vi "Vision Auto Target.vi"(11 "navX Device":T1={"Interface"={"Protocol"=enum."SERIAL", "Update Rate (4Hz-60Hz)"=4, "navX Open TypeDef"=variant}, "Notify Packet"=refnum, "Loop VI Refnum"=refnum, "Ready to Close Occurrence Refnum"=refnum} {"Interface"."Update Rate (4Hz-60Hz)" min=4 max=60 step=1}) -> ()   [LabVIEW 2015]
uses:
  NavX/navX Library v2/TypeDefs/Z900_navX_DeviceTypeDef.ctl
  NavX/navX Library v2/TypeDefs/Z900_navX_ProtocolTypeDef.ctl
  NavX/navX Library v2/TypeDefs/Z900_navX_NotifyPacketTypeDef.ctl
  NavX/navX Library v2/TypeDefs/Z900_navX_ActionTypeDef.ctl
  Team Code/Robot Global Data.vi
  <vilib>/Rock Robotics/Network Tables/NT Write Number.vi
  NavX/navX Library v2/navX Library v2.lvlib
panel:
  in  "Vertical Linear Relationship":dbl
  out "VisionVertical":cluster{"VisionGyroTarget":dbl, dbl, dbl}(graph)
  out "VisionStateDistance":enum16{"Disabled", "Enable", "Suspended", "PID"}(ring)
  in  "VeriticalOffset":dbl=0.033
  in  "Y gain":dbl=80.0
  in  "minimumVisionValue":dbl=0.45
  in  "X Gain":dbl=80.0
  in  "minimumVisionValue":dbl=0.45
  out "VisionHorizontal":cluster{"VisionGyroTarget":dbl, dbl, dbl}(graph)
  out "VisionStateAngle":enum16{"Disabled", "Enable", "Suspended", "PID"}(ring)
  in  "HorizontalOffset":dbl=0.066
  # "More positive = counter clockwise\nMore negative = clockwise"
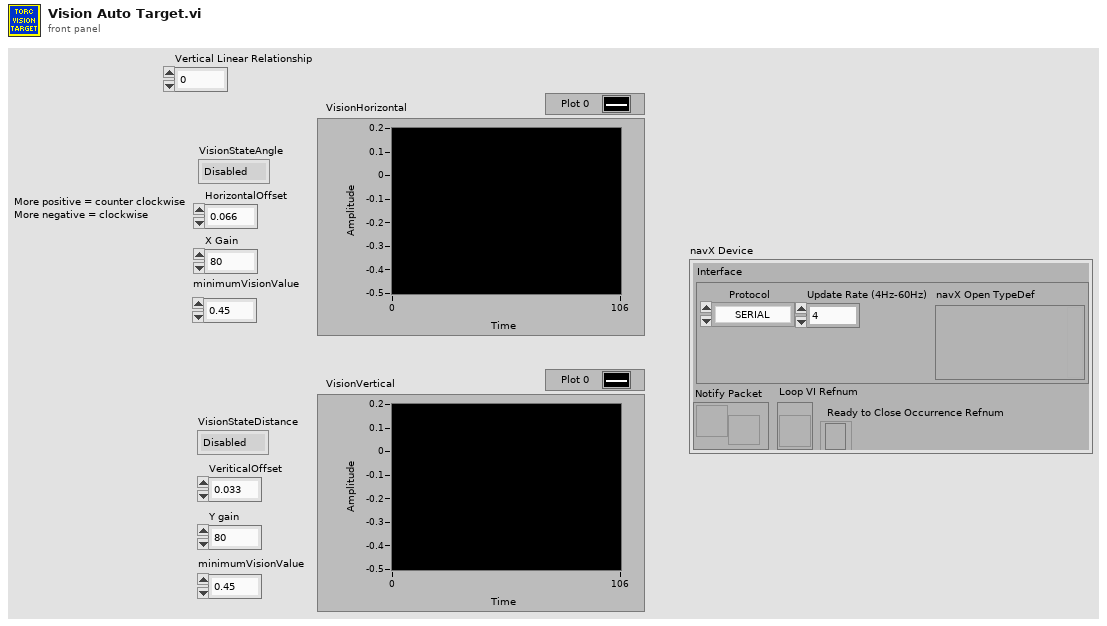
[diagram p1: front panel]
types:
  T1 = typedef "navX Library v2.lvlib/Z900_navX_DeviceTypeDef.ctl" = cluster{"Interface":cluster{"Protocol":T2, "Update Rate (4Hz-60Hz)":u8, "navX Open TypeDef":variant}, "Notify Packet":refnum<notifier>, "Loop VI Refnum":refnum<vi>, "Ready to Close Occurrence Refnum":refnum<k4>}
  T2 = typedef "navX Library v2.lvlib/Z900_navX_ProtocolTypeDef.ctl" = enum16{"SERIAL", "I2C", "SPI"}
  T3 = cluster{"Yaw":dbl, "Roll":dbl, "Pitch":dbl, "Heading":dbl, "Fused Heading":dbl}
  T4 = cluster{"Distance (ft)":dbl, "Center":cluster{dbl, dbl}, "Normalized Rect":cluster{"Numeric":dbl, "Numeric 2":dbl, "Numeric 3":dbl, "Numeric 5":dbl}}[]
  T5 = cluster{"Detected Targets[0]":cluster{"Distance (ft)":dbl, "Center":cluster{dbl, dbl}, "Normalized Rect":cluster{"Numeric":dbl, "Numeric 2":dbl, "Numeric 3":dbl, "Numeric 5":dbl}}, "Detected Targets[1]":cluster{"Distance (ft)":dbl, "Center":cluster{dbl, dbl}, "Normalized Rect":cluster{"Numeric":dbl, "Numeric 2":dbl, "Numeric 3":dbl, "Numeric 5":dbl}}, "Detected Targets[2]":cluster{"Distance (ft)":dbl, "Center":cluster{dbl, dbl}, "Normalized Rect":cluster{"Numeric":dbl, "Numeric 2":dbl, "Numeric 3":dbl, "Numeric 5":dbl}}, "Detected Targets[3]":cluster{"Distance (ft)":dbl, "Center":cluster{dbl, dbl}, "Normalized Rect":cluster{"Numeric":dbl, "Numeric 2":dbl, "Numeric 3":dbl, "Numeric 5":dbl}}, "Detected Targets[4]":cluster{"Distance (ft)":dbl, "Center":cluster{dbl, dbl}, "Normalized Rect":cluster{"Numeric":dbl, "Numeric 2":dbl, "Numeric 3":dbl, "Numeric 5":dbl}}, "Detected Targets[5]":cluster{"Distance (ft)":dbl, "Center":cluster{dbl, dbl}, "Normalized Rect":cluster{"Numeric":dbl, "Numeric 2":dbl, "Numeric 3":dbl, "Numeric 5":dbl}}, "Detected Targets[6]":cluster{"Distance (ft)":dbl, "Center":cluster{dbl, dbl}, "Normalized Rect":cluster{"Numeric":dbl, "Numeric 2":dbl, "Numeric 3":dbl, "Numeric 5":dbl}}, "Detected Targets[7]":cluster{"Distance (ft)":dbl, "Center":cluster{dbl, dbl}, "Normalized Rect":cluster{"Numeric":dbl, "Numeric 2":dbl, "Numeric 3":dbl, "Numeric 5":dbl}}, "Detected Targets[8]":cluster{"Distance (ft)":dbl, "Center":cluster{dbl, dbl}, "Normalized Rect":cluster{"Numeric":dbl, "Numeric 2":dbl, "Numeric 3":dbl, "Numeric 5":dbl}}}
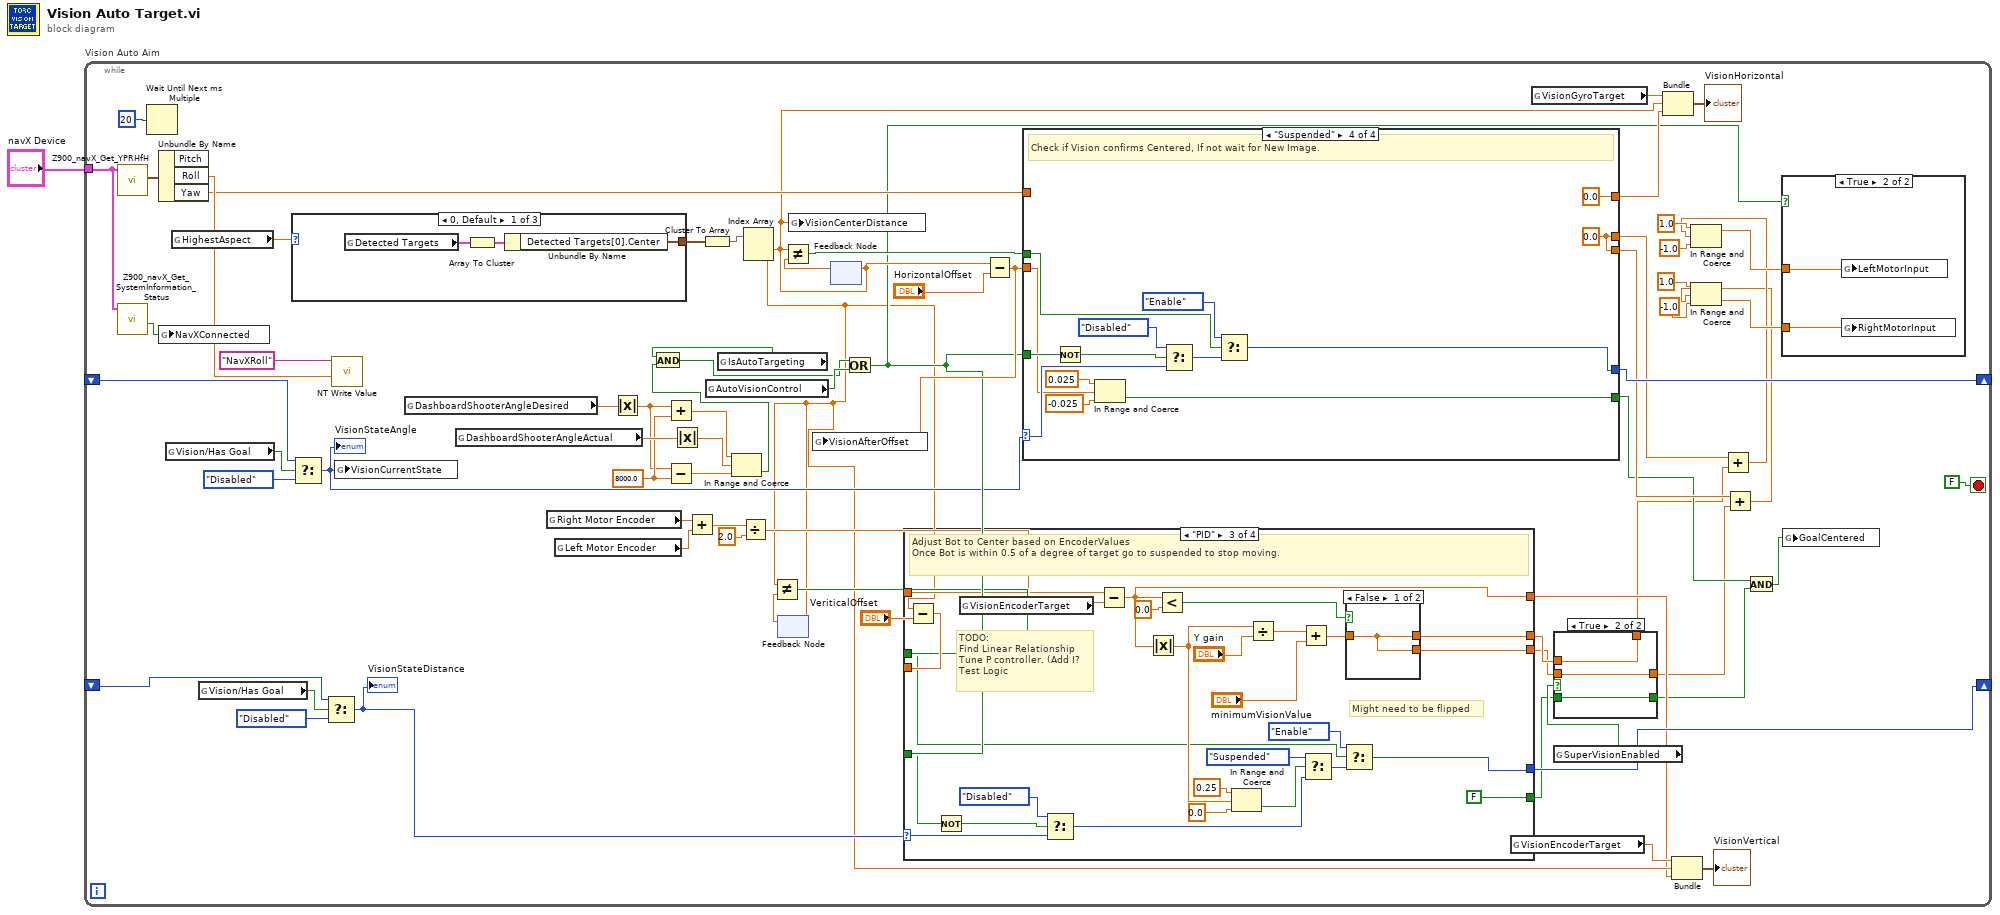
[diagram p0: block diagram]
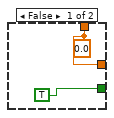
[diagram p2: hidden frame]
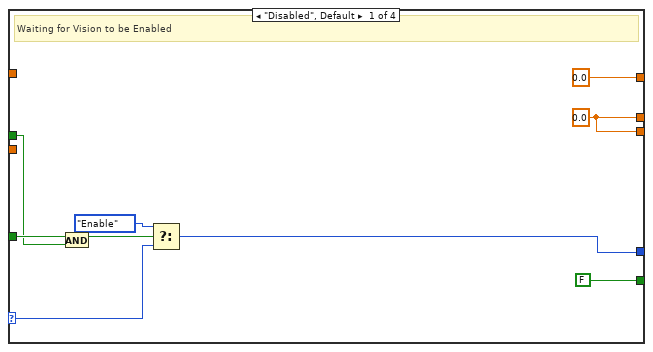
[diagram p3: hidden frame]
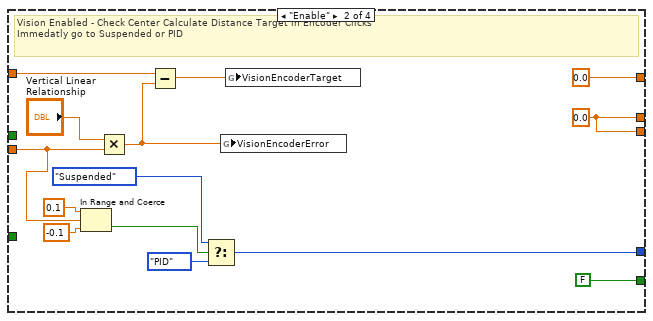
[diagram p4: hidden frame]
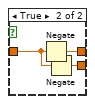
[diagram p5: hidden frame]
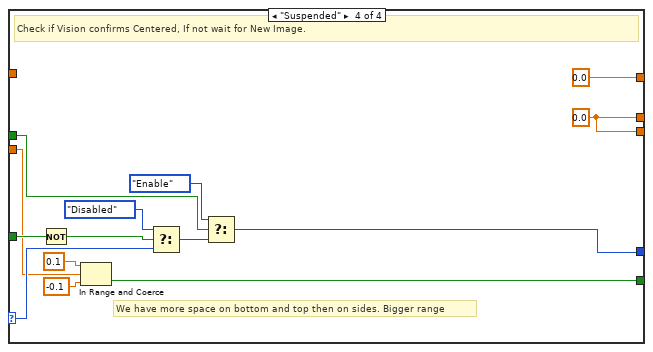
[diagram p6: hidden frame]
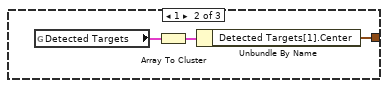
[diagram p7: hidden frame]
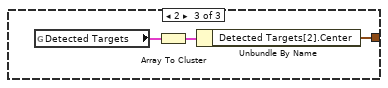
[diagram p8: hidden frame]
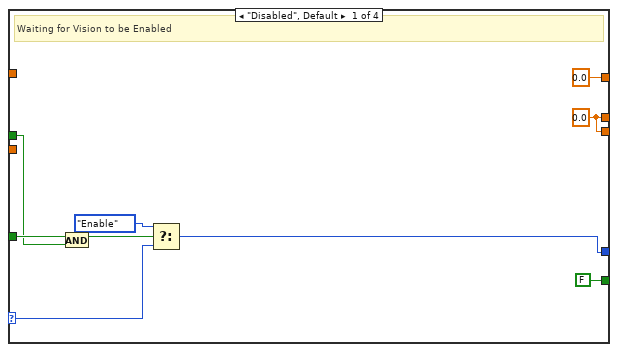
[diagram p10: hidden frame]
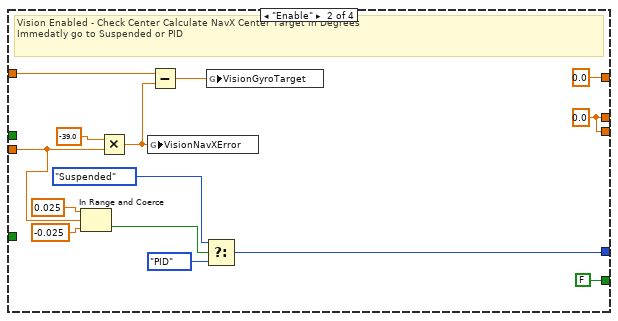
[diagram p11: hidden frame]
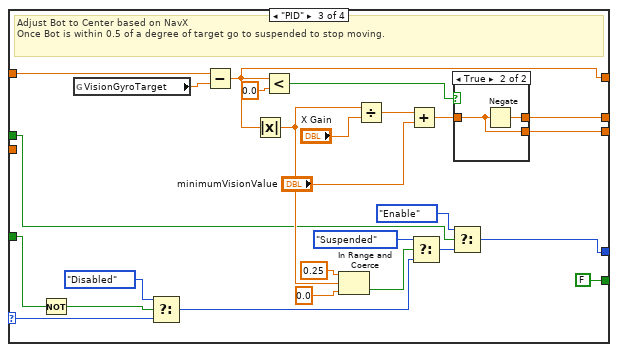
[diagram p12: hidden frame]
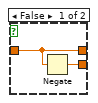
[diagram p13: hidden frame]
diagram:
  n1 = while "Vision Auto Aim" {
    tunnel: "navX Device" -> [w68]
    shift-right: [w71] -> _
    shift-left: _ -> [w54]
    shift-right: [w18] -> _
    shift-left: _ -> [w15]
    stop <- FALSE stop-if-true
    w42 = 8000.0 ("y")
    n2 = call "Z900_navX_Get_YPRHfH.vi"("navX Device"=w68) -> ("YRPHfH"=w72:T3)  [unwired: 7 in, 3 out]
    n3 = call "Z900_navX_Get_SystemInformation_Status.vi"("navX Device"=w68) -> ("Connected"=w55:bool)  [unwired: 7 in, 3 out]
    n4 = Wait Until Next ms Multiple(millisecond multiple=u32 20 ("milliseconds to wait")) -> ()  [unwired: 1 out]
    n5 = Unbundle By Name(w72) -> ("Roll"=w70:dbl, "Yaw"=w49:dbl)  [unwired: 1 out]
    n6 = global write "Robot Global Data.vi" "NavXConnected"(w55) -> ()
    n7 = global read "Robot Global Data.vi" "Vision/Has Goal"() -> (w53:bool)
    n8 = global read "Robot Global Data.vi" "HighestAspect"() -> (w51:dbl)
    n9 = global read "Robot Global Data.vi" "Vision/Has Goal"() -> (w17:bool)
    n10 = case shown="0, Default" w51 {
      tunnel: [w147 w150 w153] -> w58
      frame 0, Default {
        n11 = global read "Robot Global Data.vi" "Detected Targets"() -> (w148:T4)
        n12 = Array To Cluster(array=w148) -> (cluster=w149:T5)
        n13 = Unbundle By Name(w149) -> ("Detected Targets[0].Center"=w147:cluster{dbl, dbl})
      }
      frame 1 {
        n14 = global read "Robot Global Data.vi" "Detected Targets"() -> (w151:T4)
        n15 = Array To Cluster(array=w151) -> (cluster=w152:T5)
        n16 = Unbundle By Name(w152) -> ("Detected Targets[1].Center"=w150:cluster{dbl, dbl})
      }
      frame 2 {
        n17 = global read "Robot Global Data.vi" "Detected Targets"() -> (w154:T4)
        n18 = Array To Cluster(array=w154) -> (cluster=w155:T5)
        n19 = Unbundle By Name(w155) -> ("Detected Targets[2].Center"=w153:cluster{dbl, dbl})
      }
    }
    n20 = Select(t=w54, s=w53, f=enum16{"Disabled", "Enable", "Suspended", "PID"}."Disabled" ("t")) -> (s? t:f=w21:enum16{"Disabled", "Enable", "Suspended", "PID"})
    "VisionStateAngle" <- w21
    n21 = Select(t=w15, s=w17, f=enum16{"Disabled", "Enable", "Suspended", "PID"}."Disabled" ("t")) -> (s? t:f=w14:enum16{"Disabled", "Enable", "Suspended", "PID"})
    "VisionStateDistance" <- w14
    n22 = call-poly <vilib>:"NT Write Value.vi"("Numeric"=w70, "Name"="NavXRoll") -> ()  [unwired: 9 in, 1 out]
    n23 = global write "Robot Global Data.vi" "VisionCurrentState"(w21) -> ()
    n24 = global read "Robot Global Data.vi" "DashboardShooterAngleDesired"() -> (w44:dbl)
    n25 = global read "Robot Global Data.vi" "DashboardShooterAngleActual"() -> (w47:dbl)
    n26 = global read "Robot Global Data.vi" "Right Motor Encoder"() -> (w30:dbl)
    n27 = global read "Robot Global Data.vi" "Left Motor Encoder"() -> (w29:dbl)
    n28 = Absolute Value(x=w44) -> (abs(x)=w41:dbl)
    n29 = Add(x=w41, y=w42) -> (x+y=w46:dbl)
    n30 = Subtract(x=w41, y=w42) -> (x-y=w45:dbl)
    n31 = Absolute Value(x=w47) -> (abs(x)=w43:dbl)
    n32 = Add(x=w30, y=w29) -> (x+y=w28:dbl)
    n33 = Cluster To Array(cluster=w58) -> (array=w13:dbl[])
    n34 = global read "Robot Global Data.vi" "AutoVisionControl"() -> (w56:bool)
    n35 = global read "Robot Global Data.vi" "IsAutoTargeting"() -> (w40:bool)
    n36 = In Range and Coerce(upper limit=w46, x=w43, lower limit=w45) -> (In Range?=w39:bool)  [unwired: 1 out]
    n37 = And(x=w40, y=w39) -> (x .and. y?=w38:bool)
    n38 = Divide(x=w28, y=2.0) -> (x/y=w26:dbl)
    n39 = Index Array(array=w13) -> (element #1=w48:dbl, element #2=w11:dbl)  [unwired: 2 in]
    n40 = feedback #1() -> (w34:dbl)  [unwired: 1 in]
    n41 = Not Equal?(x=w11, y=w34) -> (x != y?=w31:bool)
    n42 = feedback-in #1(w11) -> ()
    n43 = global write "Robot Global Data.vi" "VisionCenterDistance"(w48) -> ()
    n44 = feedback-in #2(w48) -> ()
    n45 = feedback #2() -> (w57:dbl)  [unwired: 1 in]
    n46 = Not Equal?(x=w48, y=w57) -> (x != y?=w36:bool)
    n47 = Or(x=w38, y=w56) -> (x .or. y?=w35:bool)
    n48 = Subtract(x=w11, y="VeriticalOffset") -> (x-y=w32:dbl)
    n49 = case shown="\"PID\"" w14 {
      selector: w14 -> [w88 _ w104 w136]
      tunnel: w35 -> [w84 _ w107 w138]
      tunnel: [w86 w100 w109 w137] -> w18
      tunnel: w26 -> [_ w95 w116 _]
      tunnel: [FALSE FALSE FALSE w134] -> w3
      tunnel: w32 -> [_ w91 _ w133]
      tunnel: [w83 w97 w118 w146] -> w8
      tunnel: [w83 w97 w119 w146] -> w6
      tunnel: [0.0 0.0 w115 0.0] -> w9
      tunnel: w31 -> [w80 _ w103 w135]
      frame "Disabled", Default {
        w83 = 0.0
        # "Waiting for Vision to be Enabled"
        n50 = And(x=w84, y=w80) -> (x .and. y?=w81:bool)
        n51 = Select(t=enum16{"Disabled", "Enable", "Suspended", "PID"}."Enable", s=w81, f=w88) -> (s? t:f=w86:enum16{"Disabled", "Enable", "Suspended", "PID"})
      }
      frame "Enable" {
        w97 = 0.0 ("LeftMotorOutput")
        # "Vision Enabled - Check Center Calculate Distance Target in Encoder Clicks\nImmedatly go to Suspended or PID"
        n52 = In Range and Coerce(upper limit=0.1, x=w91, lower limit=-0.1) -> (In Range?=w93:bool)  [unwired: 1 out]
        n53 = Multiply(x="Vertical Linear Relationship", y=w91) -> (x*y=w94:dbl)
        n54 = Subtract(x=w95, y=w94) -> (x-y=w90:dbl)
        n55 = Select(t=enum16{"Disabled", "Enable", "Suspended", "PID"}."Suspended", s=w93, f=enum16{"Disabled", "Enable", "Suspended", "PID"}."PID" ("t")) -> (s? t:f=w100:enum16{"Disabled", "Enable", "Suspended", "PID"})
        n56 = global write "Robot Global Data.vi" "VisionEncoderError"(w94) -> ()
        n57 = global write "Robot Global Data.vi" "VisionEncoderTarget"(w90) -> ()
      }
      frame "PID" {
        # "Might need to be flipped"
        # "TODO: \nFind Linear Relationship\nTune P controller. (Add I?\nTest Logic"
        # "Adjust Bot to Center based on EncoderValues\nOnce Bot is within 0.5 of a degree of target go to suspended to stop moving."
        n58 = Not(x=w107) -> (.not. x?=w106:bool)
        n59 = global read "Robot Global Data.vi" "VisionEncoderTarget"() -> (w125:dbl)
        n60 = Select(t=enum16{"Disabled", "Enable", "Suspended", "PID"}."Disabled", s=w106, f=w104) -> (s? t:f=w105:enum16{"Disabled", "Enable", "Suspended", "PID"})
        n61 = Subtract(x=w116, y=w125) -> (x-y=w115:dbl)
        n62 = Absolute Value(x=w115) -> (abs(x)=w113:dbl)
        n63 = Less?(x=w115, y=0.0) -> (x < y?=w121:bool)
        n64 = In Range and Coerce(upper limit=0.25, x=w113, lower limit=0.0) -> (In Range?=w128:bool)  [unwired: 1 out]
        n65 = Divide(x=w113, y="Y gain") -> (x/y=w123:dbl)
        n66 = Add(x=w123, y="minimumVisionValue") -> (x+y=w120:dbl)
        n67 = Select(t=enum16{"Disabled", "Enable", "Suspended", "PID"}."Suspended", s=w128, f=w105) -> (s? t:f=w110:enum16{"Disabled", "Enable", "Suspended", "PID"})
        n68 = Select(t=enum16{"Disabled", "Enable", "Suspended", "PID"}."Enable", s=w103, f=w110) -> (s? t:f=w109:enum16{"Disabled", "Enable", "Suspended", "PID"})
        n69 = case shown="False" w121 {
          tunnel: w120 -> [w129 w131]
          tunnel: [w129 w130] -> w119
          tunnel: [w129 w132] -> w118
          frame False {
          }
          frame True {
            n70 = Negate(x=w131) -> (-x=w132:dbl)
            n71 = Negate(x=w131) -> (-x=w130:dbl)
          }
        }
      }
      frame "Suspended" {
        w146 = 0.0 ("LeftMotorOutput")
        # "We have more space on bottom and top then on sides. Bigger range"
        # "Check if Vision confirms Centered, If not wait for New Image."
        n72 = Not(x=w138) -> (.not. x?=w139:bool)
        n73 = In Range and Coerce(upper limit=0.1, x=w133, lower limit=-0.1) -> (In Range?=w134:bool)  [unwired: 1 out]
        n74 = Select(t=enum16{"Disabled", "Enable", "Suspended", "PID"}."Disabled" ("f"), s=w139, f=w136) -> (s? t:f=w141:enum16{"Disabled", "Enable", "Suspended", "PID"})
        n75 = Select(t=enum16{"Disabled", "Enable", "Suspended", "PID"}."Enable" ("f"), s=w135, f=w141) -> (s? t:f=w137:enum16{"Disabled", "Enable", "Suspended", "PID"})
      }
    }
    n76 = Subtract(x=w48, y="HorizontalOffset") -> (x-y=w37:dbl)
    n77 = global write "Robot Global Data.vi" "VisionAfterOffset"(w37) -> ()
    n78 = case shown="\"Suspended\"" w21 {
      selector: w21 -> [w166 _ w182 w214]
      tunnel: w35 -> [w162 _ w185 w216]
      tunnel: [w164 w178 w187 w215] -> w71
      tunnel: w49 -> [_ w171 w194 _]
      tunnel: [FALSE FALSE FALSE w212] -> w20
      tunnel: w37 -> [_ w167 _ w211]
      tunnel: [w161 w174 w196 w224] -> w25
      tunnel: [w161 w174 w197 w224] -> w24
      tunnel: [0.0 0.0 w193 0.0] -> w60
      tunnel: w36 -> [w158 _ w181 w213]
      frame "Disabled", Default {
        w161 = 0.0
        # "Waiting for Vision to be Enabled"
        n79 = And(x=w162, y=w158) -> (x .and. y?=w159:bool)
        n80 = Select(t=enum16{"Disabled", "Enable", "Suspended", "PID"}."Enable", s=w159, f=w166) -> (s? t:f=w164:enum16{"Disabled", "Enable", "Suspended", "PID"})
      }
      frame "Enable" {
        w174 = 0.0 ("LeftMotorOutput")
        # "Vision Enabled - Check Center Calculate NavX Center Target in Degrees\nImmedatly go to Suspended or PID"
        n81 = In Range and Coerce(upper limit=0.025, x=w167, lower limit=-0.025) -> (In Range?=w169:bool)  [unwired: 1 out]
        n82 = Multiply(x=-39.0, y=w167) -> (x*y=w170:dbl)
        n83 = global write "Robot Global Data.vi" "VisionNavXError"(w170) -> ()
        n84 = Subtract(x=w171, y=w170) -> (x-y=w173:dbl)
        n85 = Select(t=enum16{"Disabled", "Enable", "Suspended", "PID"}."Suspended", s=w169, f=enum16{"Disabled", "Enable", "Suspended", "PID"}."PID" ("t")) -> (s? t:f=w178:enum16{"Disabled", "Enable", "Suspended", "PID"})
        n86 = global write "Robot Global Data.vi" "VisionGyroTarget"(w173) -> ()
      }
      frame "PID" {
        # "Adjust Bot to Center based on NavX\nOnce Bot is within 0.5 of a degree of target go to suspended to stop moving."
        n87 = Not(x=w185) -> (.not. x?=w184:bool)
        n88 = global read "Robot Global Data.vi" "VisionGyroTarget"() -> (w203:dbl)
        n89 = Select(t=enum16{"Disabled", "Enable", "Suspended", "PID"}."Disabled", s=w184, f=w182) -> (s? t:f=w183:enum16{"Disabled", "Enable", "Suspended", "PID"})
        n90 = Subtract(x=w194, y=w203) -> (x-y=w193:dbl)
        n91 = Absolute Value(x=w193) -> (abs(x)=w191:dbl)
        n92 = Less?(x=w193, y=0.0) -> (x < y?=w199:bool)
        n93 = In Range and Coerce(upper limit=0.25, x=w191, lower limit=0.0) -> (In Range?=w206:bool)  [unwired: 1 out]
        n94 = Divide(x=w191, y="X Gain") -> (x/y=w201:dbl)
        n95 = Add(x=w201, y="minimumVisionValue") -> (x+y=w198:dbl)
        n96 = Select(t=enum16{"Disabled", "Enable", "Suspended", "PID"}."Suspended", s=w206, f=w183) -> (s? t:f=w188:enum16{"Disabled", "Enable", "Suspended", "PID"})
        n97 = Select(t=enum16{"Disabled", "Enable", "Suspended", "PID"}."Enable", s=w181, f=w188) -> (s? t:f=w187:enum16{"Disabled", "Enable", "Suspended", "PID"})
        n98 = case shown="True" w199 {
          tunnel: w198 -> [w208 w209]
          tunnel: [w207 w209] -> w197
          tunnel: [w208 w210] -> w196
          frame False {
            n99 = Negate(x=w208) -> (-x=w207:dbl)
          }
          frame True {
            n100 = Negate(x=w209) -> (-x=w210:dbl)
          }
        }
      }
      frame "Suspended" {
        w224 = 0.0 ("LeftMotorOutput")
        # "Check if Vision confirms Centered, If not wait for New Image."
        n101 = Not(x=w216) -> (.not. x?=w217:bool)
        n102 = In Range and Coerce(upper limit=0.025, x=w211, lower limit=-0.025) -> (In Range?=w212:bool)  [unwired: 1 out]
        n103 = Select(t=enum16{"Disabled", "Enable", "Suspended", "PID"}."Disabled" ("f"), s=w217, f=w214) -> (s? t:f=w219:enum16{"Disabled", "Enable", "Suspended", "PID"})
        n104 = Select(t=enum16{"Disabled", "Enable", "Suspended", "PID"}."Enable" ("f"), s=w213, f=w219) -> (s? t:f=w215:enum16{"Disabled", "Enable", "Suspended", "PID"})
      }
    }
    n105 = global read "Robot Global Data.vi" "VisionEncoderTarget"() -> (w12:dbl)
    n106 = global read "Robot Global Data.vi" "VisionGyroTarget"() -> (w61:dbl)
    n107 = global read "Robot Global Data.vi" "SuperVisionEnabled"() -> (w4:bool)
    n108 = case shown="True" w4 {
      tunnel: w8 -> [_ w79]
      tunnel: [w76 w79] -> w7
      tunnel: w6 -> [_ w78]
      tunnel: [w76 w78] -> w5
      tunnel: w3 -> [_ w77]
      tunnel: [TRUE w77] -> w2
      frame False {
        w76 = 0.0 ("LeftMotorOutput")
      }
      frame True {
      }
    }
    n109 = Bundle("VisionGyroTarget"=w61, w48, w60) -> (→"VisionHorizontal":cluster{"VisionGyroTarget":dbl, dbl, dbl})  [unwired: 1 in]
    n110 = Bundle("VisionEncoderTarget"=w12, w11, w9) -> (→"VisionVertical":cluster{"VisionEncoderTarget":dbl, dbl, dbl})  [unwired: 1 in]
    n111 = Add(x=w25, y=w7) -> (x+y=w23:dbl)
    n112 = In Range and Coerce(upper limit=1.0, x=w23, lower limit=-1.0) -> (coerced(x)=w63:dbl)  [unwired: 1 out]
    n113 = Add(x=w24, y=w5) -> (x+y=w22:dbl)
    n114 = In Range and Coerce(upper limit=1.0, x=w22, lower limit=-1.0) -> (coerced(x)=w62:dbl)  [unwired: 1 out]
    n115 = And(x=w20, y=w2) -> (x .and. y?=w19:bool)
    n116 = case shown="True" w35 {
      tunnel: w62 -> [_ w156]
      tunnel: w63 -> [_ w157]
      frame False {
      }
      frame True {
        n117 = global write "Robot Global Data.vi" "LeftMotorInput"(w157) -> ()
        n118 = global write "Robot Global Data.vi" "RightMotorInput"(w156) -> ()
      }
    }
    n119 = global write "Robot Global Data.vi" "GoalCentered"(w19) -> ()
  }
